vi "MovemotorMengXYMain.vi"(4 "Serial number":i32, 6 "Joystick axis":i32, 8 "error in (no error)":errorcluster, 9 "MAX":sgl, 10 "MIN":sgl, 11 "Automation Refnum in":refnum<k7>) -> (0 "error out":errorcluster, 2 "Automation Refnum out":refnum<k7>, 3 "XorYPosition":sgl)   [LabVIEW 2014]
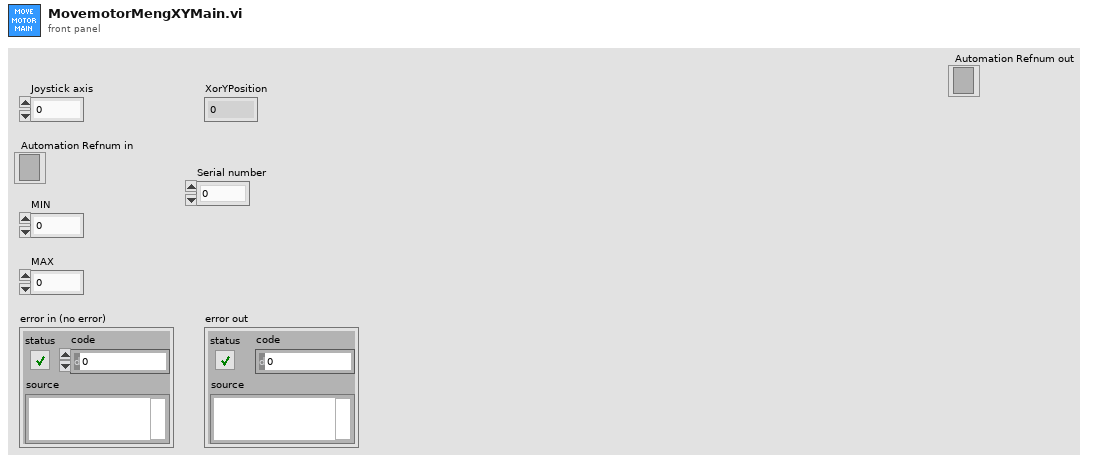
[diagram p1: front panel]
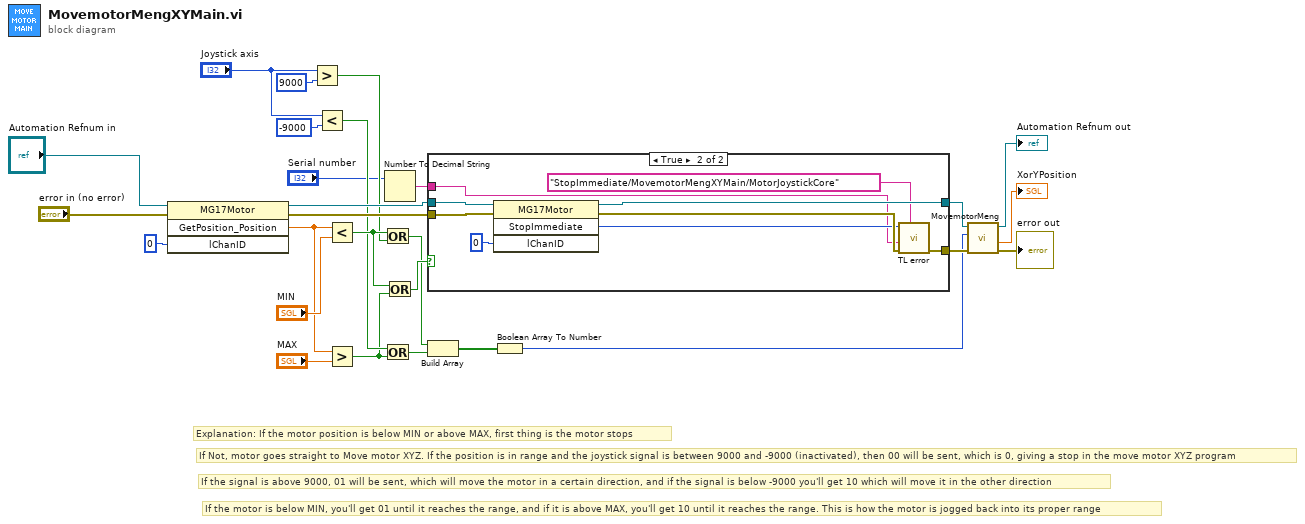
[diagram p0: block diagram]
diagram:
  # "If the motor is below MIN, you'll get 01 until it reaches the range, and if it is above MAX, you'll get 10 until it reaches the range. This is how the motor is jogged back into its proper range"
  # "If the signal is above 9000, 01 will be sent, which will move the motor in a certain direction, and if the signal is below -9000 you'll get 10 which will move it in the other direction"
  # "If Not, motor goes straight to Move motor XYZ. If the position is in range and the joystick signal is between 9000 and -9000 (inactivated), then 00 will be sent, which is 0, giving a stop in the move motor XYZ program"
  # "Explanation: If the motor position is below MIN or above MAX, first thing is the motor stops"
  n1 = invoke class="MG17Motor" method="GetPosition_Position"(reference="Automation Refnum in", error in="error in (no error)", "lChanID"=0) -> (reference out=w23:refnum<k7>, error out=w22:errorcluster, "GetPosition_Position"=w13:sgl)  [unwired: 1 in, 1 out]
  n2 = Greater?(x="Joystick axis", y=9000) -> (0:w15:bool)
  n3 = Less?(x="Joystick axis", y=-9000) -> (x < y?=w12:bool)
  n4 = Less?(x=w13, y="MIN") -> (x < y?=w20:bool)
  n5 = Greater?(x=w13, y="MAX") -> (0:w1:bool)
  n6 = Or(x=w20, y=w15) -> (x .or. y?=w16:bool)
  n7 = Or(x=w12, y=w1) -> (x .or. y?=w17:bool)
  n8 = Number To Decimal String(number="Serial number") -> (decimal integer string=w2:string)  [unwired: 1 in]
  n9 = Or(x=w20, y=w1) -> (x .or. y?=w21:bool)
  n10 = case shown="True" w21 {
    tunnel: w23 -> [w29 w38]
    tunnel: w22 -> [w28 w37]
    tunnel: [w28 w33] -> w25
    tunnel: [w29 w36] -> w24
    tunnel: w2 -> [_ w31]
    frame False {
    }
    frame True {
      n11 = invoke class="MG17Motor" method="StopImmediate"(reference=w38, error in=w37, "lChanID"=0) -> (reference out=w36:refnum<k7>, error out=w34:errorcluster, "StopImmediate"=w32:i32)  [unwired: 1 in, 1 out]
      n12 = call "TL error.vi"("Input string"="StopImmediate/MovemotorMengXYMain/MotorJoystickCore", "error in (no error)"=w34, "Serial number of motor"=w31, "Return Code"=w32) -> ("error out"=w33:errorcluster)  [unwired: 7 in]
    }
  }
  n13 = Build Array(w16, w17) -> (w7:bool[])
  n14 = Boolean Array To Number(Boolean array=w7) -> (number=w9:u32)
  n15 = call "MovemotorMeng.vi"("error in (no error)"=w25, "Input"=w9, "Automation Refnum in"=w24) -> ("error out"=→"error out":errorcluster, "Position"=→"XorYPosition":sgl, "Automation Refnum out"=→"Automation Refnum out":refnum<k7>)  [unwired: 6 in]
